vi "Elapse_Time_string.vi"(11 "y":timestamp format="%<%.3X\n%Y/%m/%d>T") -> (3 "Elased Time(S)":string)   [LabVIEW 2017]
panel:
  out "min":dbl
  out "error out":errorcluster
  in  "error in (no error)":errorcluster
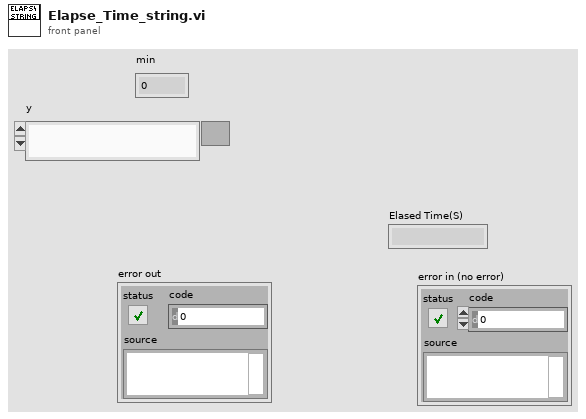
[diagram p1: front panel]
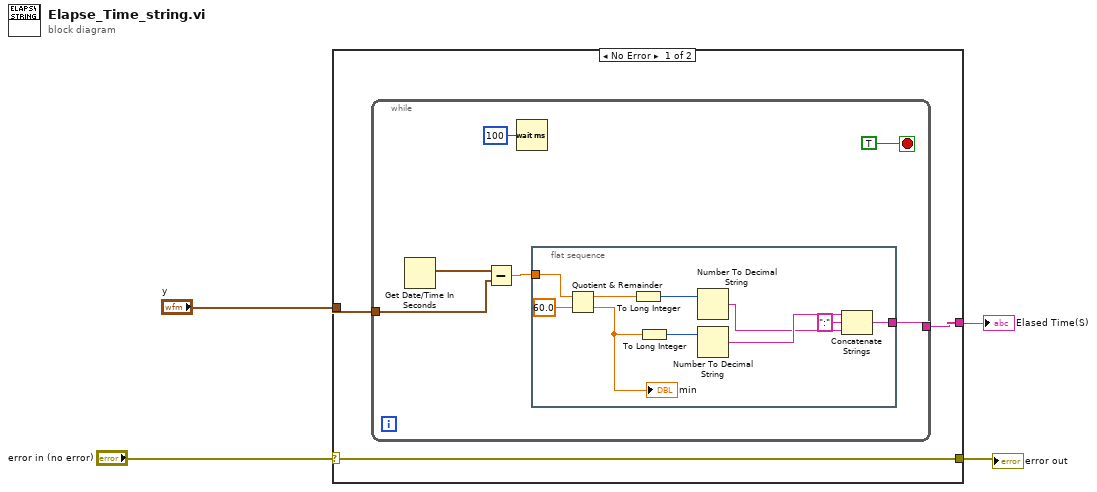
[diagram p0: block diagram]
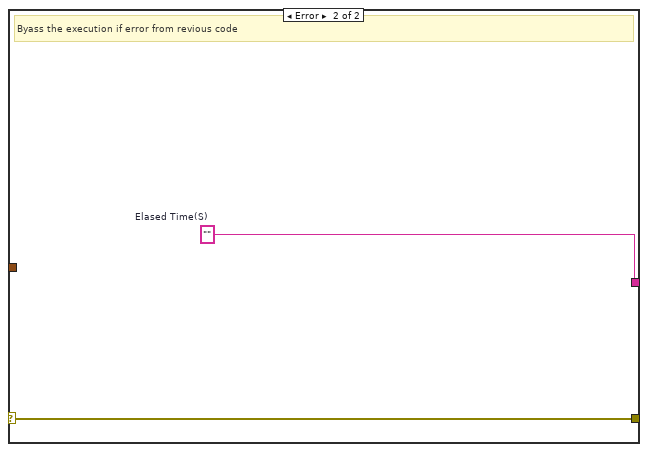
[diagram p2: hidden frame]
diagram:
  n1 = case shown="No Error" "error in (no error)" {
    selector: "error in (no error)" -> [w7 w25]
    tunnel: [w7 w25] -> w3
    tunnel: [w6 w24] -> w2
    tunnel: "y" -> [w5 _]
    frame No Error {
      n2 = while {
        tunnel: [w11] -> w6
        tunnel: w5 -> [w8]
        stop <- TRUE stop-if-true
        n3 = Get Date/Time In Seconds() -> (seconds since 1Jan1904=w10:timestamp)
        n4 = Subtract(x=w10, y=w8) -> (x-y=w9:dbl)
        n5 = Wait (ms)(milliseconds to wait=u32 100) -> ()  [unwired: 1 out]
        n6 = flat-sequence {
          tunnel: [w15] -> w11
          tunnel: w9 -> [w14]
          frame #0 {
            n7 = Quotient & Remainder(x=w14, y=60.0) -> (x-y*floor(x/y)=w21:dbl, floor(x/y)=w22:dbl)
            "min" <- w22
            n8 = To Long Integer(number=w21) -> (32bit integer=w17:i32)
            n9 = To Long Integer(number=w22) -> (32bit integer=w16:i32)
            n10 = Number To Decimal String(number=w17) -> (decimal integer string=w19:string)  [unwired: 1 in]
            n11 = Number To Decimal String(number=w16) -> (decimal integer string=w20:string)  [unwired: 1 in]
            n12 = Concatenate Strings(w20, ":" ("string"), w19) -> (w15:string)
          }
        }
      }
    }
    frame Error {
      w24 = ""  # Elased Time(S)
      # "Byass the execution if error from revious code"
    }
  }
  "Elased Time(S)" <- w2
  "error out" <- w3
